vi "set_I_one_channel.vi"() -> ()   [LabVIEW 2017]
uses:
  types/channels_enum.ctl
panel:
  in  "value_control":bool=TRUE
  out "error out":errorcluster
  out "VISA resource name 2":refnum<visa-resource-name>
  in  "curr":dbl=0.001 min=0.001 max=0.999
  in  "channel":T1=enum."1"
  in  "error in (no error)":errorcluster
  in  "VISA resource name":refnum<visa-resource-name>
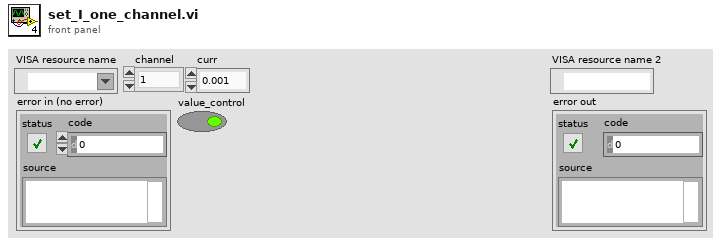
[diagram p1: front panel]
types:
  T1 = typedef "channels_enum.ctl" = enum16{"0", "1", "2"}
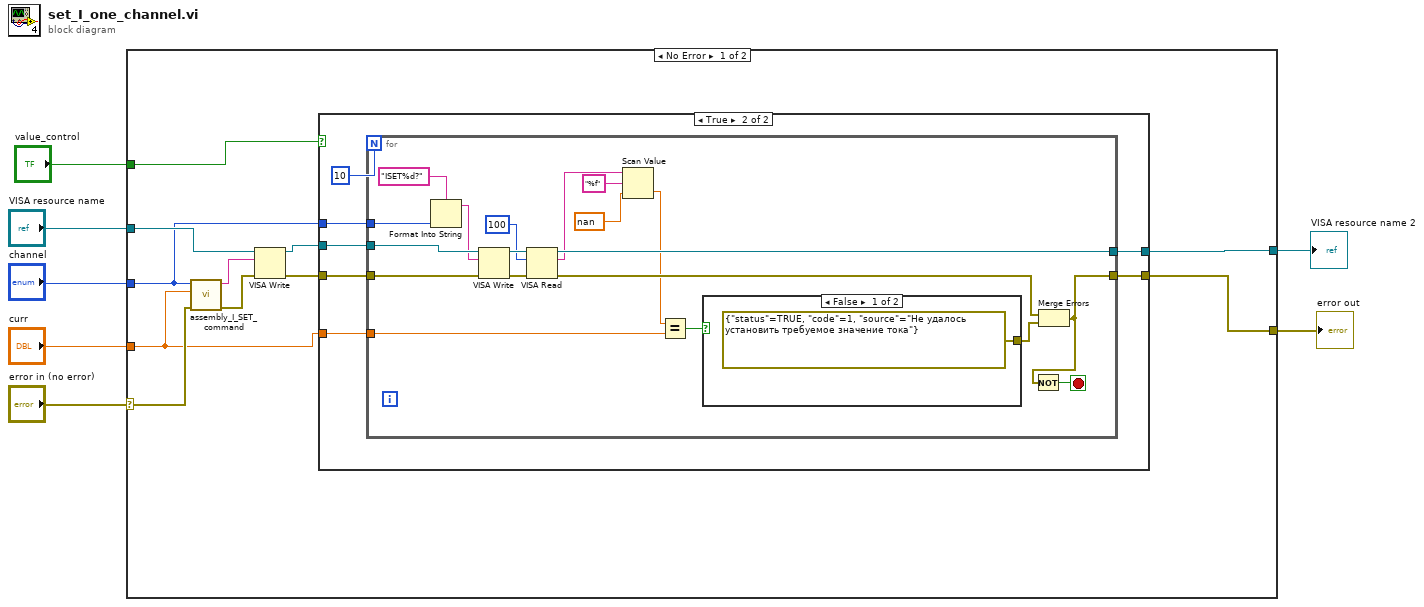
[diagram p0: block diagram]
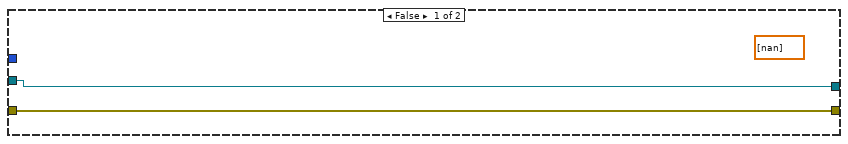
[diagram p2: hidden frame]
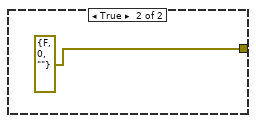
[diagram p3: hidden frame]
diagram:
  n1 = case shown="No Error" "error in (no error)" {
    selector: "error in (no error)" -> [w9 w50]
    tunnel: "VISA resource name" -> [w18 w49]
    tunnel: [w14 w49] -> w6
    tunnel: [w13 w50] -> w5
    tunnel: "value_control" -> [w12 _]
    tunnel: "channel" -> [w11 _]
    tunnel: "curr" -> [w8 _]
    frame No Error {
      n2 = call "assembly_I_SET_command.vi"("error_in"=w9, "curr"=w8, "channel"=w11) -> ("error_out"=w10:errorcluster, "command"=w17:string)  [unwired: 7 in]
      n3 = VISA Write(VISA resource name=w18, write buffer=w17, error in (no error)=w10) -> (VISA resource name out=w16:refnum<visa-resource-name>, error out=w15:errorcluster)  [unwired: 1 out]
      n4 = case shown="True" w12 {
        tunnel: w16 -> [w20 w27]
        tunnel: w15 -> [w19 w26]
        tunnel: [w20 w24] -> w14
        tunnel: [w19 w23] -> w13
        tunnel: w8 -> [_ w22]
        tunnel: w11 -> [_ w21]
        frame False {
          (unwired) dbl[] [nan]
        }
        frame True {
          n5 = for {
            N: 10 -> [_]
            tunnel: w27 -> [w46]
            tunnel: w26 -> [w45]
            tunnel: [w41] -> w24
            tunnel: [w33] -> w23
            tunnel: w22 -> [w37]
            tunnel: w21 -> [w30]
            stop <- w34 stop-if-true
            n6 = Format Into String(format string="ISET%d?" ("write buffer"), w30) -> (resulting string=w29:string)  [unwired: 2 in, 1 out]
            n7 = VISA Write(VISA resource name=w46, write buffer=w29, error in (no error)=w45) -> (VISA resource name out=w44:refnum<visa-resource-name>, error out=w43:errorcluster)  [unwired: 1 out]
            n8 = VISA Read(VISA resource name=w44, byte count=u32 100, error in (no error)=w43) -> (VISA resource name out=w41:refnum<visa-resource-name>, read buffer=w39:string, error out=w35:errorcluster)  [unwired: 1 out]
            n9 = Scan Value(string=w39, format string="%f", default (0 dbl)=nan) -> (value=w28:dbl)  [unwired: 1 out]
            n10 = Equal?(x=w28, y=w37) -> (x = y?=w38:bool)
            n11 = case shown="False" w38 {
              tunnel: [errorcluster {"status"=TRUE, "code"=1, "source"="Не удалось установить требуемое значение тока"} ("error constant") errorcluster {"status"=FALSE, "code"=0, "source"=""} ("error constant")] -> w36
              frame False {
              }
              frame True {
              }
            }
            n12 = Merge Errors(w35, w36) -> (w33:errorcluster)
            n13 = Not(x=w33) -> (.not. x?=w34:bool)
          }
        }
      }
    }
    frame Error {
    }
  }
  "VISA resource name 2" <- w6
  "error out" <- w5
